vi "CREATE_LOGGING_STRING.vi"(10 "Array":dbl[](array[numeric]), 11 "String in":string) -> (3 "String out":string)   [LabVIEW 2016]
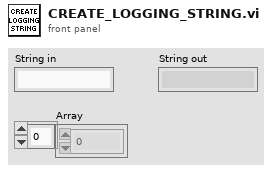
[diagram p1: front panel]
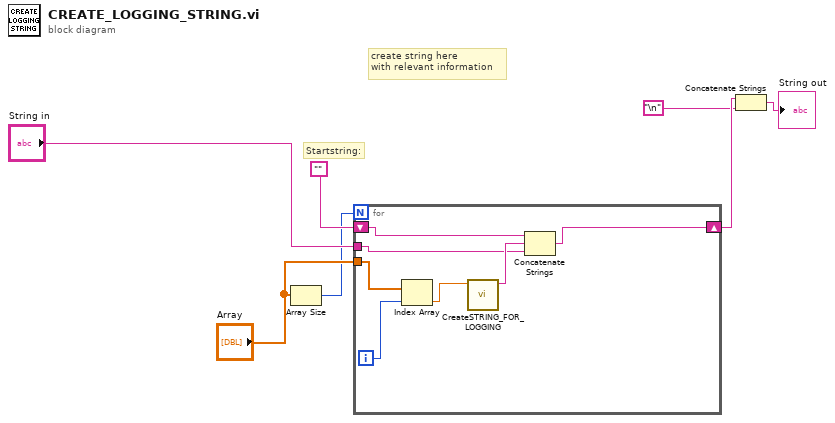
[diagram p0: block diagram]
diagram:
  # "Startstring:"
  # "create string here \nwith relevant information"
  n1 = Array Size(array="Array") -> (size(s)=w4:i32)
  n2 = for {
    N: w4 -> [_]
    tunnel: "Array" -> [w13]
    tunnel: "String in" -> [w10]
    shift-right: [w8] -> w3
    shift-left: "" -> [w9]
    i -> [w14]
    n3 = Index Array(array=w13, index=w14) -> (element=w12:dbl)
    n4 = call "CreateSTRING_FOR_LOGGING.vi"("input DBL"=w12) -> ("String"=w11:string)  [unwired: 10 in]
    n5 = Concatenate Strings(w9, w11, w10) -> (w8:string)
  }
  n6 = Concatenate Strings(w3, "\n") -> (→"String out":string)
